vi "Send Items To Target.vi"(4 "Remove Items on PC":bool, 5 "Local Path":string, 6 "wait for reply (T)":bool=TRUE, 7 "Path on Target":string, 8 "error in":errorcluster, 9 "TransferOptions":refnum<class "FileTransferOptions.lvclass">, 10 "Transfer Type":T4, 11 "Module ID":i32=-1) -> (0 "error out":errorcluster, 1 "timed out?":bool, 2 "Reply Payload":T1)   [LabVIEW 2015, in "LV-WinSCP.lvlib"]
doc: "This request allows transferring a file or the content of an entire folder from the local PC to the remote target.\nFile transfer status might take longer than the module timeout. A broadcast is then also fired with the transfer status when it finishes. Therefore, asking for a reply is optional.\nA connection to the target (valid session) must be done before using this request.\n_____\nCreated using DQMH Event Scripter 6.1.0.128."
uses:
  LV-WinSCP.lvlib
  Transfer Type.ctl
  Classes/FileTransferOptions/FileTransferOptions.lvclass
  Send Items To Target (Reply Payload)--cluster.ctl
  Classes/FileTransfer/FileAndDestination.ctl
  Classes/FileTransfer/TransferExceptionDescription.ctl
  Send Items To Target Argument--cluster.ctl
  Classes/FileTransfer/FileTransfer.lvclass
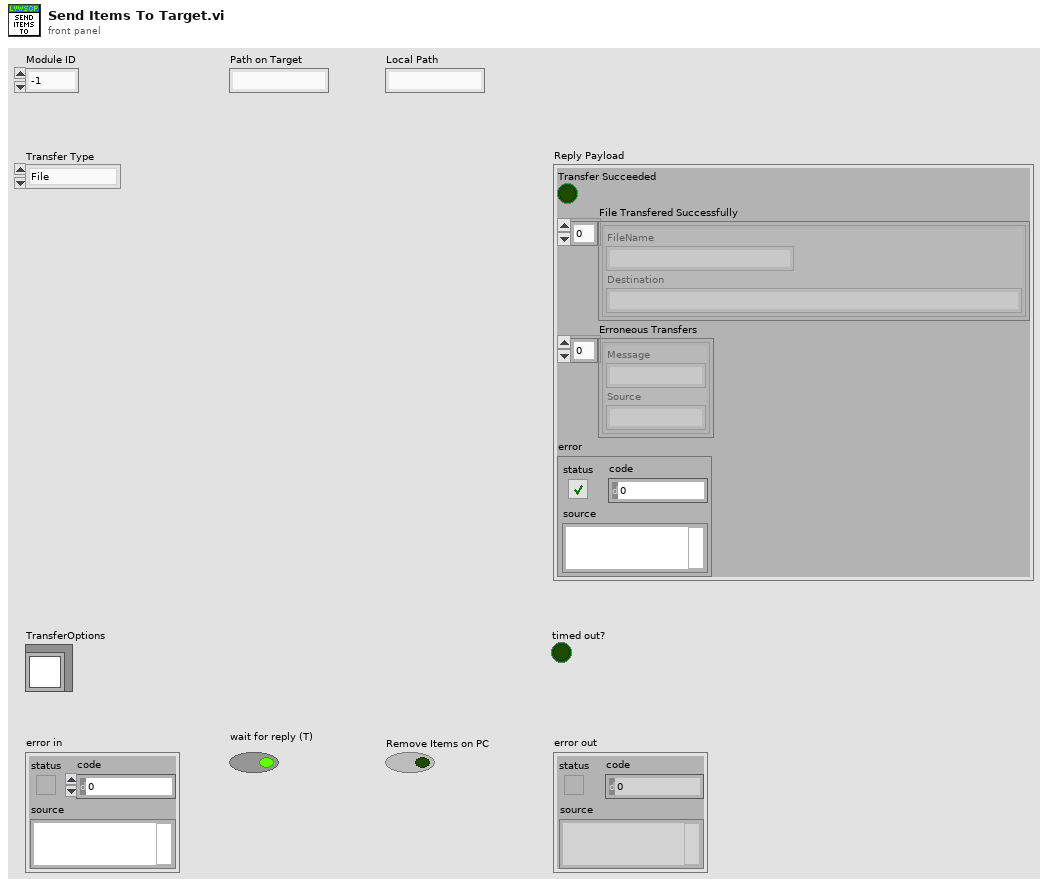
[diagram p1: front panel]
types:
  T1 = typedef "LV-WinSCP.lvlib/Send Items To Target (Reply Payload)--cluster.ctl" = cluster{"Transfer Succeeded":bool, "File Transfered Successfully":T2[], "Erroneous Transfers":T3[], "error":errorcluster}
  T2 = typedef "WinSCP.lvlib/FileTransfer.lvclass/FileAndDestination.ctl" = cluster{"FileName":string, "Destination":string}
  T3 = typedef "WinSCP.lvlib/FileTransfer.lvclass/TransferExceptionDescription.ctl" = cluster{"Message":string, "Source":string}
  T4 = typedef "LV-WinSCP.lvlib/Transfer Type.ctl" = enum16{"File", "Folder"}
  T5 = typedef "LV-WinSCP.lvlib/Send Items To Target Argument--cluster.ctl" = cluster{"Module ID":i32, "Transfer Type":T4, "TransferOptions":refnum<class "FileTransferOptions.lvclass">, "Path on Target":string, "Local Path":string, "Remove Items on PC":bool, "Wait Notifier":refnum<notifier>, "wait for reply":bool}
  T6 = typedef "LV-WinSCP.lvlib/Request Events--cluster.ctl" = cluster{"Stop Module":refnum<user-event>, "Show Panel":refnum<user-event>, "Hide Panel":refnum<user-event>, "Show Diagram":refnum<user-event>, "Get Module Execution Status":refnum<user-event>, "Initialize Session":refnum<user-event>, "Close Session":refnum<user-event>, "List Directory":refnum<user-event>, "Get Items From Target":refnum<user-event>, "Execute Command On Target":refnum<user-event>, "Send Items To Target":refnum<user-event>}
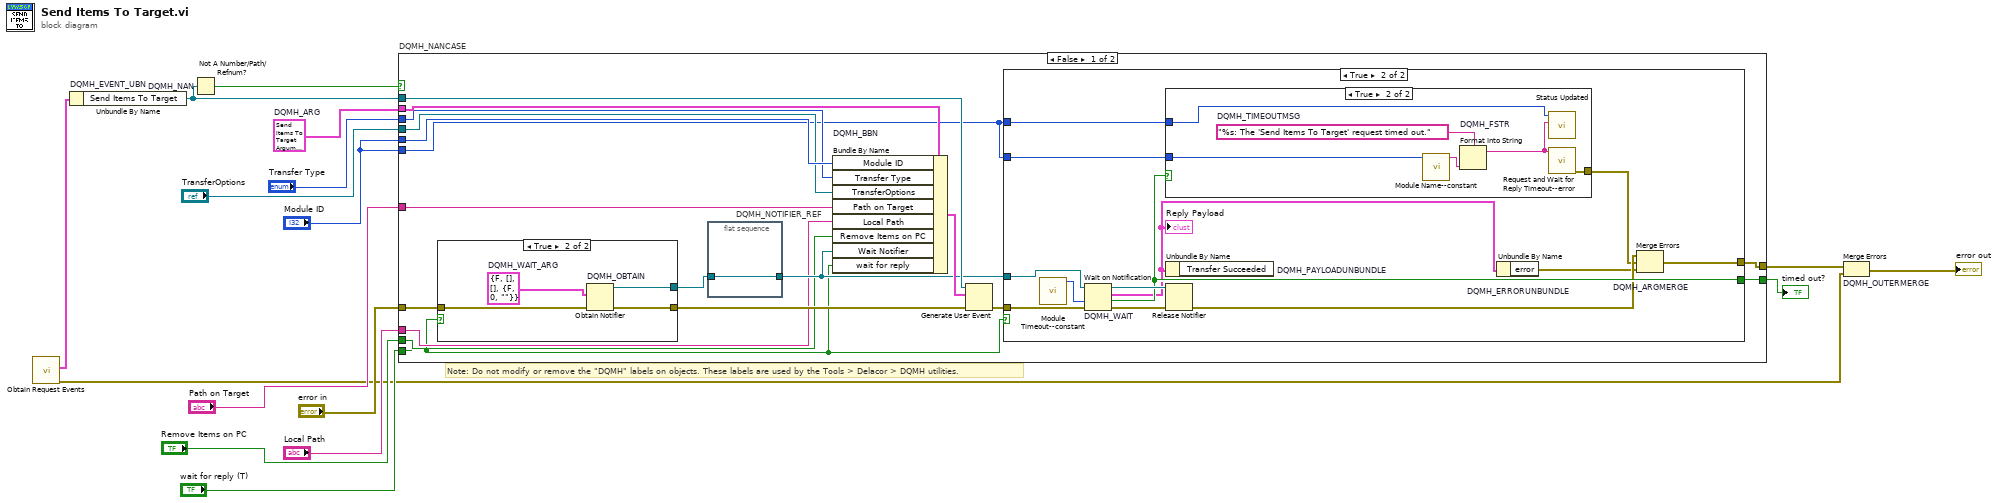
[diagram p0: block diagram]
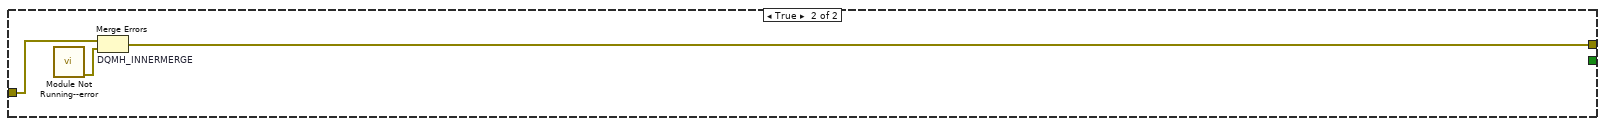
[diagram p5: hidden frame]
diagram:
  w10 = T5 {"Module ID"=-1, "Transfer Type"=enum."File", "TransferOptions"=refnum, "Path on Target"="", "Local Path"="", "Remove Items on PC"=FALSE, "Wait Notifier"=refnum, "wait for reply"=FALSE}  # DQMH_ARG
  # "Note: Do not modify or remove the \"DQMH\" labels on objects. These labels are used by the Tools > Delacor > DQMH utilities."
  n1 = call "Obtain Request Events.vi"() -> ("error out"=w2:errorcluster, "LV-WinSCP Request Events"=w1:T6)  [unwired: 10 in]
  n2 = Unbundle By Name "DQMH_EVENT_UBN"(w1) -> ("Send Items To Target"=w14:refnum<user-event>)
  n3 = Not A Number/Path/Refnum? "DQMH_NAN"(number/path/refnum=w14) -> (NaN/Path/Refnum?=w13:bool)
  n4 = case "DQMH_NANCASE" shown="False" w13 {
    tunnel: "error in" -> [w34 w63]
    tunnel: w14 -> [w32 _]
    tunnel: [w29 w62] -> w11
    tunnel: [w30 _] -> w12
    tunnel: w10 -> [w25 _]
    tunnel: "Module ID" -> [w24 _]
    tunnel: "Transfer Type" -> [w23 _]
    tunnel: "TransferOptions" -> [w22 _]
    tunnel: "Path on Target" -> [w21 _]
    tunnel: "Local Path" -> [w20 _]
    tunnel: "Remove Items on PC" -> [w19 _]
    tunnel: "Module ID" -> [w18 _]
    tunnel: "wait for reply (T)" -> [w17 _]
    frame False {
      n5 = case shown="True" w17 {
        tunnel: w34 -> [w56 w60]
        tunnel: [w56 w59] -> w31
        tunnel: [_ w57] -> w27
        frame False {
        }
        frame True {
          w58 = T1 {"Transfer Succeeded"=FALSE, "File Transfered Successfully"=[], "Erroneous Transfers"=[], "error"={"status"=FALSE, "code"=0, "source"=""}}  # DQMH_WAIT_ARG
          n6 = Obtain Notifier "DQMH_OBTAIN"(notification data type=w58, error in (no error)=w60) -> (notifier out=w57:refnum<notifier>, error out=w59:errorcluster)  [unwired: 2 in, 1 out]
        }
      }
      n7 = flat-sequence "DQMH_NOTIFIER_REF" {
        tunnel: w27 -> [w35]
        tunnel: [w35] -> w26
        frame #0 {
        }
      }
      n8 = Bundle By Name "DQMH_BBN"(cluster=w25, "Module ID"=w24, "Transfer Type"=w23, "TransferOptions"=w22, "Path on Target"=w21, "Local Path"=w20, "Remove Items on PC"=w19, "Wait Notifier"=w26, "wait for reply"=w17) -> (w28:T5)
      n9 = Generate User Event(user event=w32, event data cluster=w28, error in=w31) -> (error out=w33:errorcluster)  [unwired: 1 in, 1 out]
      n10 = case shown="True" w17 {
        tunnel: w33 -> [w36 w49]
        tunnel: w26 -> [_ w48]
        tunnel: [_ w46] -> w30
        tunnel: [w36 w45] -> w29
        tunnel: w18 -> [_ w38]
        tunnel: w18 -> [_ w37]
        frame False {
        }
        frame True {
          n11 = call "Module Timeout--constant.vi"() -> ("Module Timeout"=w39:i32)  [unwired: 11 in]
          n12 = Wait on Notification "DQMH_WAIT"(notifier=w48, timeout in ms (-1)=w39, error in (no error)=w49) -> (notifier out=w47:refnum<notifier>, notification=w40:T1, timed out?=w46:bool, error out=w44:errorcluster)  [unwired: 1 in]
          "Reply Payload" <- w40
          n13 = case shown="True" w46 {
            tunnel: [_ w53] -> w41
            tunnel: w38 -> [_ w51]
            tunnel: w37 -> [_ w50]
            frame False {
            }
            frame True {
              w55 = "%s: The 'Send Items To Target' request timed out."  # DQMH_TIMEOUTMSG
              n14 = call "Module Name--constant.vi"("Module ID"=w50) -> ("Module Name"=w52:string)  [unwired: 10 in]
              n15 = Format Into String "DQMH_FSTR"(format string=w55, w52) -> (resulting string=w54:string)  [unwired: 2 in, 1 out]
              n16 = call "Status Updated.vi"("Status"=w54, "Module ID"=w51) -> ()  [unwired: 9 in, 1 out]
              n17 = call "Request and Wait for Reply Timeout--error.vi"("Error Message"=w54) -> ("error out"=w53:errorcluster)  [unwired: 10 in]
            }
          }
          n18 = Unbundle By Name "DQMH_PAYLOADUNBUNDLE"(w40) -> ()  [unwired: 1 out]
          n19 = Release Notifier(notifier=w47, error in (no error)=w44) -> (error out=w43:errorcluster)  [unwired: 1 in, 2 out]
          n20 = Unbundle By Name "DQMH_ERRORUNBUNDLE"(w40) -> ("error"=w42:errorcluster)
          n21 = Merge Errors "DQMH_ARGMERGE"(w43, w41, w42) -> (w45:errorcluster)
        }
      }
    }
    frame True {
      n22 = call "Module Not Running--error.vi"() -> ("error out"=w61:errorcluster)  [unwired: 11 in]
      n23 = Merge Errors "DQMH_INNERMERGE"(w63, w61) -> (w62:errorcluster)
    }
  }
  "timed out?" <- w12
  n24 = Merge Errors "DQMH_OUTERMERGE"(w11, w2) -> (→"error out":errorcluster)
